vi "Write Value.vi"(8 "error in (no error)":errorcluster, 10 "Value":variant, 11 "Promise in":refnum<class "Promise.lvclass">) -> (0 "error out":errorcluster, 3 "Promise out":refnum<class "Promise.lvclass">)   [LabVIEW 2017, in "Promise Future.lvlib" / "Promise.lvclass"]
uses:
  Promise.lvclass
  E:/Promise/Promise/Future/Future.lvclass
  Future/Future.lvclass
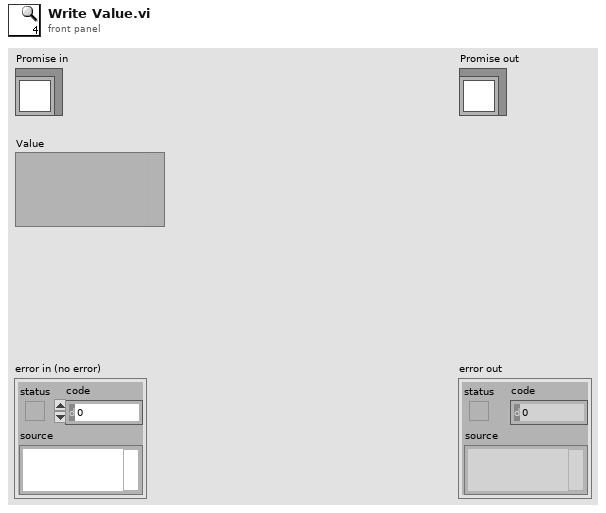
[diagram p1: front panel]
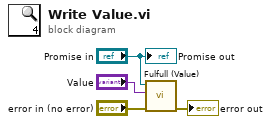
[diagram p0: block diagram]
diagram:
  n1 = call "Fulfull (Value).vi"("error in (no error)"="error in (no error)", "Value"="Value", "Future in"="Promise in") -> ("error out"=→"error out":errorcluster)  [unwired: 8 in]
  "Promise out" <- "Promise in"
